vi "LstOpenOscilloscope.vi"(8 "error in (no error)":errorcluster, 9 "dwSerialNumber in":u32) -> (0 "error out":errorcluster, 1 "dwSerialNumber out":u32, 3 "hDevice":u32)   [LabVIEW 2018, in "LibTiePie.lvlib"]
uses:
  LibTiePie.lvlib
  LabViewHS4/libtiepie.dll
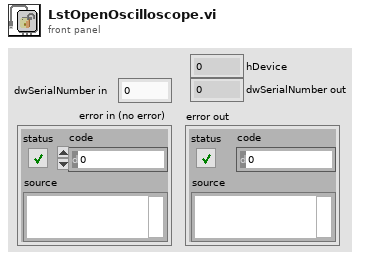
[diagram p1: front panel]
types:
  T1 = enum32{"Reserved1", "Product ID", "Index", "Reserved3", "Serial"}
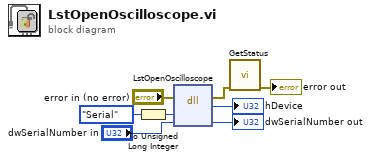
[diagram p0: block diagram]
diagram:
  n1 = To Unsigned Long Integer(number=T1."Serial" ("Indentifier")) -> (unsigned 32bit integer=w5:u32)
  n2 = dll-call lib="C:/Users/cwaha/Documents/LabViewHS4/libtiepie.dll" fn="LstOpenOscilloscope"(error in="error in (no error)", "arg1"=w5, "arg2"="dwSerialNumber in") -> (error out=w2:errorcluster, "return type"=→"hDevice":u32, "arg2"=→"dwSerialNumber out":u32)  [unwired: 3 in, 1 out]
  n3 = call "GetStatus.vi"("error in (no error)"=w2) -> ("error out"=→"error out":errorcluster)  [unwired: 10 in]
